vi "SRS 400 Read.vi"(2 "Parameters":dbl[](array[numeric]) format="%.3e", 3 "Instrument Address":refnum<visa-resource-name>) -> (0 "Stop":bool, 1 "Data":dbl[](array[numeric]))   [LabVIEW 2025]
doc: "Author: Scott Hannahs <sth@magnet.fsu.edu>\n\nThis software is licensed for use under the “MIT License\"\nCopyright (c) 2025 Scott Hannahs, sth@sth@magnet.sthnet.net\n\nPermission is hereby granted, free of charge, to any person obtaining a copy of this software and associated documentation files (the \"Software\"), to deal in the Software without restriction, including without limitation the rights to use, copy, modify, merge, publish, distribute, sublicense, and/or sell copies of the Software, and to permit persons to whom the Software is furnished to do so, subject to the following conditions: The above copyright notice and this permission notice shall be included in all copies or substantial portions of the Software.\n\nTHE SOFTWARE IS PROVIDED \"AS IS\", WITHOUT WARRANTY OF ANY KIND, EXPRESS OR IMPLIED, INCLUDING BUT NOT LIMITED TO THE WARRANTIES OF MERCHANTABILITY, FITNESS FOR A PARTICULAR PURPOSE AND NONINFRINGEMENT. IN NO EVENT SHALL THE AUTHORS OR COPYRIGHT HOLDERS BE LIABLE FOR ANY CLAIM, DAMAGES OR OTHER LIABILITY, WHETHER IN AN ACTION OF CONTRACT, TORT OR OTHERWISE, ARISING FROM, OUT OF OR IN CONNECTION WITH THE SOFTWARE OR THE USE OR OTHER DEALINGS IN THE SOFTWARE."
panel:
  # "Parameter"
  # "Value"
  # "Function"
  # "Asynchronous mode\nSynchronous mode\nCount A only\nCounts A and B"
  # "0\n1\n0\n1"
  # "0\n0\n1\n1"
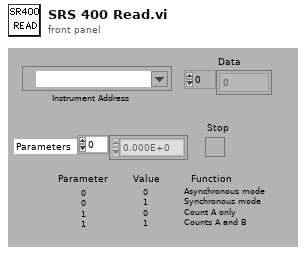
[diagram p1: front panel]
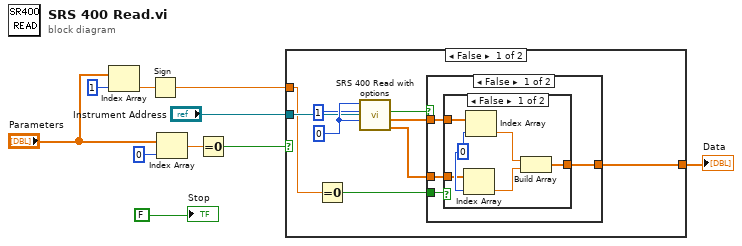
[diagram p0: block diagram]
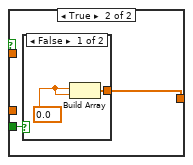
[diagram p3: hidden frame]
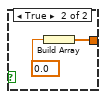
[diagram p4: hidden frame]
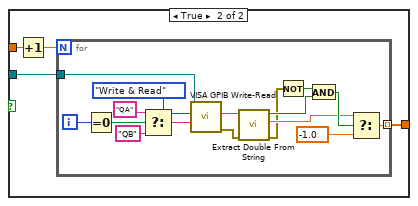
[diagram p5: hidden frame]
diagram:
  n1 = Index Array(array="Parameters", index=1) -> (element=w4:dbl)
  n2 = Sign(1:w4) -> (0:w2:dbl)
  n3 = Index Array(array="Parameters", index=0) -> (element=w6:dbl)
  n4 = Equal To 0?(x=w6) -> (x = 0?=w5:bool)
  n5 = case shown="False" w5 {
    tunnel: "Instrument Address" -> [w14 w40]
    tunnel: w2 -> [w11 w39]
    tunnel: [w13 w37] -> w3
    frame False {
      w18 = 0
      n6 = Equal To 0?(x=w11) -> (x = 0?=w12:bool)
      n7 = call "SRS 400 Read with options.vi"("Instrument Address"=w14, "dwell time"=w18, "# periods"=1, "count mode\n(a,b for t:0)"=w18) -> ("'B' data"=w17:dbl[], "'A' data"=w16:dbl[], "error"=w19:bool)  [unwired: 1 in]
      n8 = case shown="False" w19 {
        tunnel: [w23 w32] -> w13
        tunnel: w17 -> [w22 _]
        tunnel: w16 -> [w21 _]
        tunnel: w12 -> [w20 w31]
        frame False {
          n9 = case shown="False" w20 {
            tunnel: w21 -> [w29 w30]
            tunnel: w22 -> [w27 _]
            tunnel: [w24 w30] -> w23
            frame False {
              w28 = 0
              n10 = Index Array(array=w27, index=w28) -> (element=w25:dbl)
              n11 = Index Array(array=w29, index=w28) -> (element=w26:dbl)
              n12 = Build Array(w26, w25) -> (w24:dbl[])
            }
            frame True {
            }
          }
        }
        frame True {
          n13 = case shown="False" w31 {
            tunnel: [w34 w35] -> w32
            frame False {
              w33 = 0.0
              n14 = Build Array(w33, w33) -> (w34:dbl[])
            }
            frame True {
              n15 = Build Array(0.0) -> (w35:dbl[])
            }
          }
        }
      }
    }
    frame True {
      n16 = Increment(x=w39) -> (x+1=w38:dbl)
      n17 = for {
        N: w38 -> [_]
        tunnel: w40 -> [w43]
        tunnel: [w44] -> w37 mode=indexing
        i -> [w56]
        n18 = Equal To 0?(x=w56) -> (x = 0?=w45:bool)
        n19 = Select(t="QA", s=w45, f="QB") -> (s? t:f=w46:string)
        n20 = call "VISA GPIB Write-Read.vi"("Command"=w46, "Action"=enum16{"Write", "Read", "Write & Read"}."Write & Read", "VISA resource name"=w43) -> ("error out"=w42:errorcluster, "String Returned"=w50:string)  [unwired: 5 in, 2 out]
        n21 = call "Extract Double From String.vi"("error in"=w42, "string"=w50) -> ("error out"=w41:errorcluster, "floating pt. number"=w54:dbl, "valid"=w51:bool)  [unwired: 2 in, 1 out]
        n22 = Not(x=w41) -> (.not. x?=w52:bool)
        n23 = And(x=w52, y=w51) -> (x .and. y?=w55:bool)
        n24 = Select(t=w54, s=w55, f=-1.0) -> (s? t:f=w44:dbl)
      }
    }
  }
  "Data" <- w3
  "Stop" <- FALSE
